vi "Exercise3.vi"() -> ()   [LabVIEW 2019]
uses:
  <vilib>/Utility/error.llb/DialogType.ctl
  <vilib>/DAQmx/read.llb/DAQmx Read (Counter DBL 1Chan 1Samp).vi
  <vilib>/DAQmx/read.llb/DAQmx Read (Digital Bool 1Line 1Point).vi
  <vilib>/DAQmx/write.llb/DAQmx Write (Analog DBL 1Chan 1Samp).vi
  <vilib>/DAQmx/create/channels.llb/DAQmx Create Channel (AO-Voltage-Basic).vi
  <vilib>/DAQmx/create/channels.llb/DAQmx Create Channel (DI-Digital Input).vi
  <vilib>/DAQmx/create/channels.llb/DAQmx Create Channel (CI-Count Edges).vi
  <vilib>/DAQmx/miscellaneous.llb/DAQmx Fill In Error Info.vi
panel:
  out "high ticks":u32
  out "Numeric":u32
  in  "DAQmx Physical Channel":tag
  out "Bottom":bool
  out "Right":bool
  out "Left":bool
  out "Top":bool
  in  "Switch Left":tag="Dev1/ai0"
  in  "Switch Right":tag="Dev1/ai0"
  in  "Switch Top":tag="Dev1/ai0"
  in  "Switch Bottom":tag="Dev1/ai0"
  in  "Motor Stop":bool
  in  "Motor 1":dbl(slide) caption="Motor 1 (Rx - right)" scale=-10.0..10.0
  in  "Motor Left Physical Channel":tag="Dev1/ai0"
  in  "Motor 2":dbl(slide) caption="Motor 2 (Lx - left)" scale=-10.0..10.0
  in  "Maximum voltage 2":dbl
  in  "Minimum Voltage":dbl
  in  "Motor Right Physical Channel":tag="Dev1/ai0"
  in  "stop 2":bool
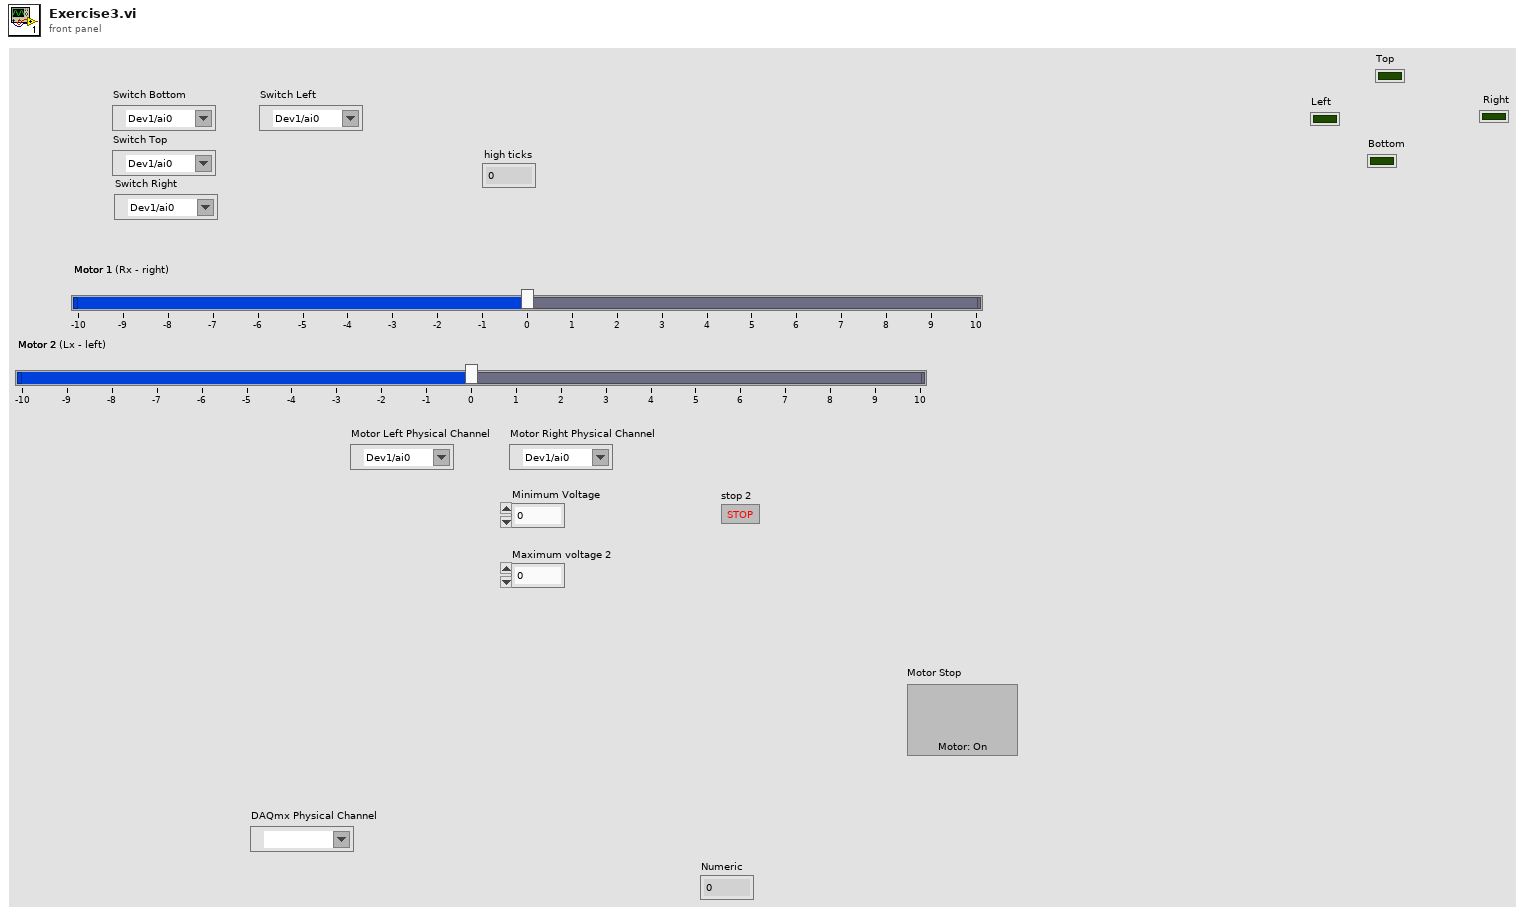
[diagram p1: front panel]
types:
  T1 = typedef "DialogType.ctl" = u16
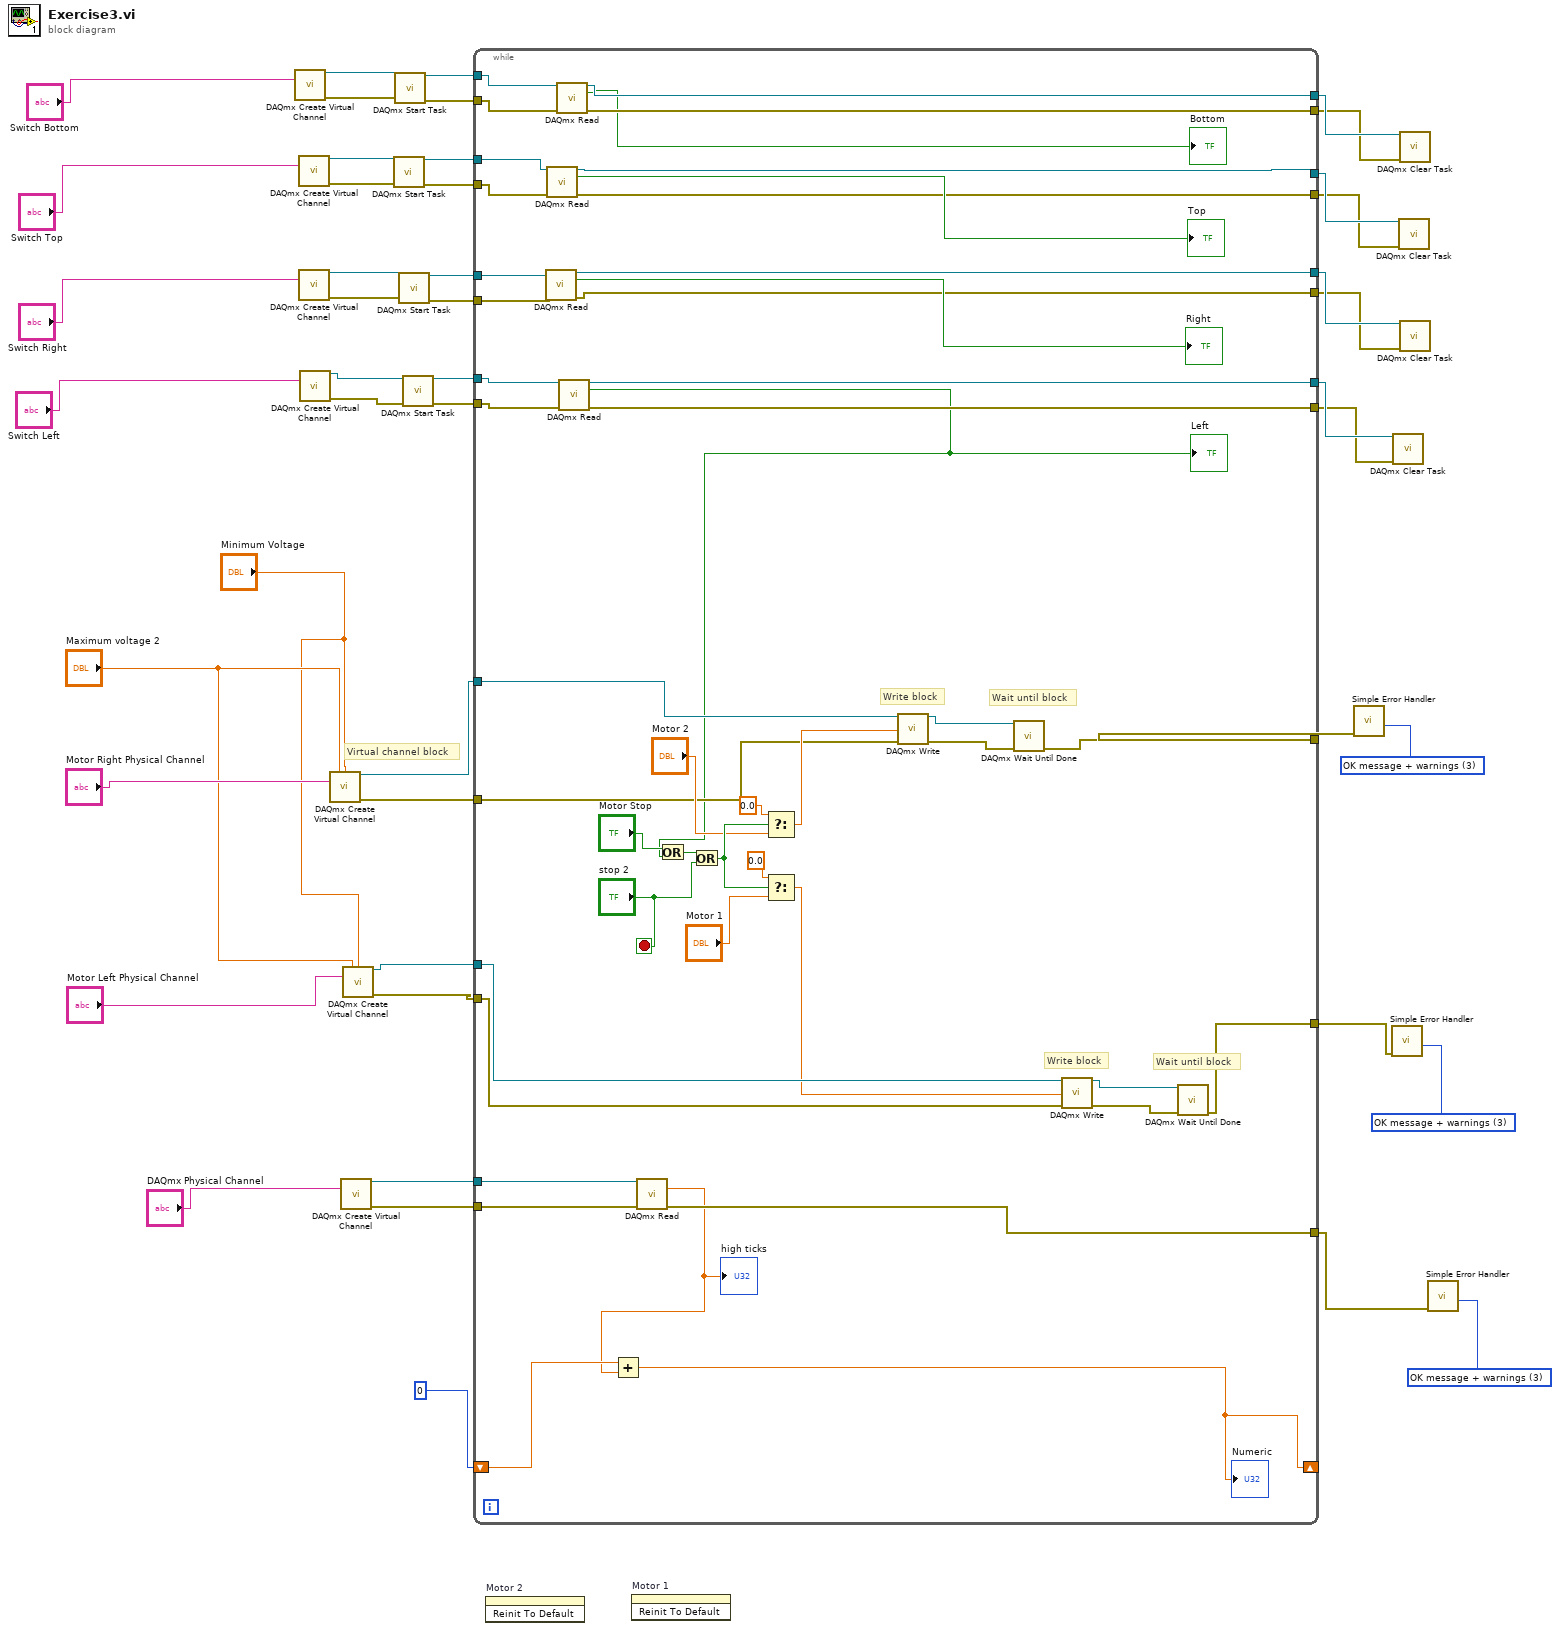
[diagram p0: block diagram]
diagram:
  w3 = T1 3 items=["no dialog", "OK message", "continue or stop message", "OK message + warnings", "continue/stop + warnings"] ("type of dialog (OK msg:1)")
  w38 = T1 3 items=["no dialog", "OK message", "continue or stop message", "OK message + warnings", "continue/stop + warnings"] ("type of dialog (OK msg:1)")
  w46 = T1 3 items=["no dialog", "OK message", "continue or stop message", "OK message + warnings", "continue/stop + warnings"] ("type of dialog (OK msg:1)")
  # "Virtual channel block"
  n1 = call-poly <vilib>:"DAQmx Create Virtual Channel.vi"("lines"="Switch Bottom") -> ("task out"=w32:refnum<k21>, "error out"=w31:errorcluster)  [unwired: 13 in]
  n2 = call-poly <vilib>:"DAQmx Create Virtual Channel.vi"("lines"="Switch Top") -> ("task out"=w30:refnum<k21>, "error out"=w29:errorcluster)  [unwired: 13 in]
  n3 = call-poly <vilib>:"DAQmx Create Virtual Channel.vi"("lines"="Switch Right") -> ("task out"=w28:refnum<k21>, "error out"=w27:errorcluster)  [unwired: 13 in]
  n4 = call-poly <vilib>:"DAQmx Create Virtual Channel.vi"("lines"="Switch Left") -> ("task out"=w26:refnum<k21>, "error out"=w25:errorcluster)  [unwired: 13 in]
  n5 = call-poly <vilib>:"DAQmx Create Virtual Channel.vi"("maximum value"="Maximum voltage 2", "minimum value"="Minimum Voltage", "physical channels"="Motor Right Physical Channel") -> ("task out"=w45:refnum<k21>, "error out"=w8:errorcluster)  [unwired: 11 in]
  n6 = call-poly <vilib>:"DAQmx Create Virtual Channel.vi"("counter"="DAQmx Physical Channel") -> ("task out"=w4:refnum<k21>, "error out"=w5:errorcluster)  [unwired: 13 in]
  n7 = call-poly <vilib>:"DAQmx Create Virtual Channel.vi"("maximum value"="Maximum voltage 2", "minimum value"="Minimum Voltage", "physical channels"="Motor Left Physical Channel") -> ("task out"=w39:refnum<k21>, "error out"=w7:errorcluster)  [unwired: 11 in]
  n8 = call <vilib>:"DAQmx Start Task.vi"("task/channels in"=w30, "error in"=w29) -> ("task out"=w23:refnum<k21>, "error out"=w21:errorcluster)  [unwired: 12 in]
  n9 = call <vilib>:"DAQmx Start Task.vi"("task/channels in"=w32, "error in"=w31) -> ("task out"=w24:refnum<k21>, "error out"=w22:errorcluster)  [unwired: 12 in]
  n10 = call <vilib>:"DAQmx Start Task.vi"("task/channels in"=w28, "error in"=w27) -> ("task out"=w19:refnum<k21>, "error out"=w20:errorcluster)  [unwired: 12 in]
  n11 = call <vilib>:"DAQmx Start Task.vi"("task/channels in"=w26, "error in"=w25) -> ("task out"=w18:refnum<k21>, "error out"=w17:errorcluster)  [unwired: 12 in]
  n12 = while {
    tunnel: w45 -> [w92]
    tunnel: [w89] -> w44
    tunnel: w39 -> [w86]
    tunnel: [w85] -> w37
    tunnel: w24 -> [w76]
    tunnel: w23 -> [w75]
    tunnel: w22 -> [w74]
    tunnel: w21 -> [w69]
    tunnel: w20 -> [w72]
    tunnel: w19 -> [w73]
    tunnel: w18 -> [w71]
    tunnel: w17 -> [w70]
    tunnel: [w68] -> w16
    tunnel: [w67] -> w14
    tunnel: [w66] -> w12
    tunnel: [w65] -> w10
    tunnel: [w64] -> w15
    tunnel: [w61] -> w13
    tunnel: [w59] -> w11
    tunnel: [w58] -> w9
    tunnel: w8 -> [w57]
    tunnel: w7 -> [w56]
    tunnel: w5 -> [w54]
    tunnel: w4 -> [w55]
    tunnel: [w53] -> w2
    shift-right: [w50] -> _
    shift-left: 0 -> [w52]
    stop <- "stop 2" stop-if-true
    # "Wait until block"
    # "Write block"
    # "Wait until block"
    # "Write block"
    n13 = call-poly <vilib>:"DAQmx Read.vi"("task/channels in"=w73, "error in"=w72) -> ("task out"=w66:refnum<k21>, "data"=→"Right":bool, "error out"=w59:errorcluster)  [unwired: 11 in]
    n14 = call-poly <vilib>:"DAQmx Read.vi"("task/channels in"=w75, "error in"=w69) -> ("task out"=w67:refnum<k21>, "data"=→"Top":bool, "error out"=w61:errorcluster)  [unwired: 11 in]
    n15 = call-poly <vilib>:"DAQmx Read.vi"("task/channels in"=w76, "error in"=w74) -> ("task out"=w68:refnum<k21>, "data"=→"Bottom":bool, "error out"=w64:errorcluster)  [unwired: 11 in]
    n16 = call-poly <vilib>:"DAQmx Read.vi"("task/channels in"=w71, "error in"=w70) -> ("task out"=w65:refnum<k21>, "data"=w47:bool, "error out"=w58:errorcluster)  [unwired: 11 in]
    "Left" <- w47
    n17 = call-poly <vilib>:"DAQmx Read.vi"("task/channels in"=w55, "error in"=w54) -> ("data"=w51:dbl, "error out"=w53:errorcluster)  [unwired: 11 in, 1 out]
    "high ticks" <- w51
    n18 = Add(x=w52, y=w51) -> (x+y=w50:dbl)
    "Numeric" <- w50
    n19 = Or(x="Motor Stop", y=w47) -> (x .or. y?=w48:bool)
    n20 = Or(x=w48, y="stop 2") -> (x .or. y?=w79:bool)
    n21 = Select(t=0.0 ("s? t:f"), s=w79, f="Motor 2") -> (s? t:f=w77:dbl)
    n22 = Select(t=0.0 ("s? t:f"), s=w79, f="Motor 1") -> (s? t:f=w81:dbl)
    n23 = call-poly <vilib>:"DAQmx Write.vi"("task/channels in"=w92, "data"=w77, "error in"=w57) -> ("task out"=w91:refnum<k21>, "error out"=w90:errorcluster)  [unwired: 10 in, 1 out]
    n24 = call <vilib>:"DAQmx Wait Until Done.vi"("task/channels in"=w91, "error in"=w90) -> ("error out"=w89:errorcluster)  [unwired: 12 in, 1 out]
    n25 = call-poly <vilib>:"DAQmx Write.vi"("task/channels in"=w86, "data"=w81, "error in"=w56) -> ("task out"=w88:refnum<k21>, "error out"=w87:errorcluster)  [unwired: 10 in, 1 out]
    n26 = call <vilib>:"DAQmx Wait Until Done.vi"("task/channels in"=w88, "error in"=w87) -> ("error out"=w85:errorcluster)  [unwired: 12 in, 1 out]
  }
  n27 = invoke on="Motor 2" class="Slide (strict)" method="Reinit To Default"() -> ()  [unwired: 3 in, 3 out]
  n28 = invoke on="Motor 1" class="Slide (strict)" method="Reinit To Default"() -> ()  [unwired: 3 in, 3 out]
  n29 = call <vilib>:"Simple Error Handler.vi"("type of dialog (OK msg:1)"=w46, "error in (no error)"=w44) -> ()  [unwired: 3 in, 5 out]
  n30 = call <vilib>:"Simple Error Handler.vi"("type of dialog (OK msg:1)"=w38, "error in (no error)"=w37) -> ()  [unwired: 3 in, 5 out]
  n31 = call <vilib>:"DAQmx Clear Task.vi"("task in"=w10, "error in"=w9) -> ()  [unwired: 13 in, 1 out]
  n32 = call <vilib>:"DAQmx Clear Task.vi"("task in"=w14, "error in"=w13) -> ()  [unwired: 13 in, 1 out]
  n33 = call <vilib>:"DAQmx Clear Task.vi"("task in"=w16, "error in"=w15) -> ()  [unwired: 13 in, 1 out]
  n34 = call <vilib>:"DAQmx Clear Task.vi"("task in"=w12, "error in"=w11) -> ()  [unwired: 13 in, 1 out]
  n35 = call <vilib>:"Simple Error Handler.vi"("type of dialog (OK msg:1)"=w3, "error in (no error)"=w2) -> ()  [unwired: 3 in, 5 out]
